vi "Scalar Destroy.vi"(8 "error in (no error)":errorcluster, 11 "Scalar DVR in":refnum<data-value>) -> (0 "error out":errorcluster)   [LabVIEW 2010, in "MDSplus.lvlib"]
uses:
  <vilib>/MDSplus/Library/MDSplus.lvlib
  <vilib>/MDSplus/Classes/Data_Class/Scalar_Class/Scalar.lvclass
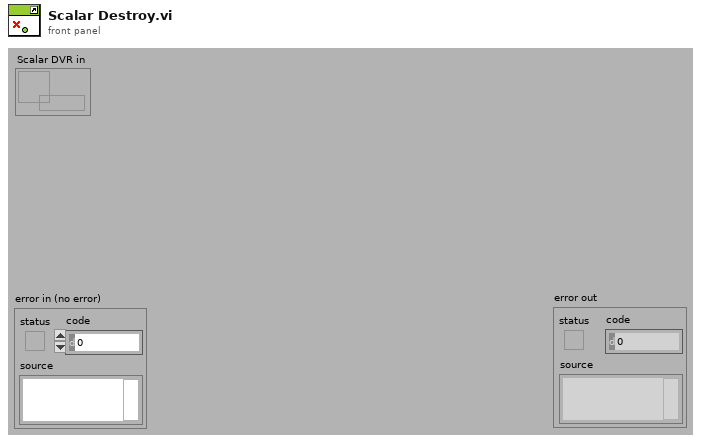
[diagram p1: front panel]
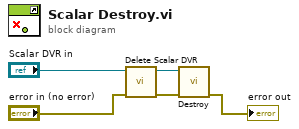
[diagram p0: block diagram]
diagram:
  n1 = call <vilib>:"Delete Scalar DVR.vi"("error in (no error)"="error in (no error)", "Scalar DVR in"="Scalar DVR in") -> ("error out"=w2:errorcluster, "Scalar out"=w3:refnum<class "Scalar.lvclass">)  [unwired: 8 in]
  n2 = call-dynamic "Destroy.vi"("error in (no error)"=w2, "Scalar in"=w3) -> ("error out"=→"error out":errorcluster)  [unwired: 9 in]
